vi "Moving Average.vi"(0 "Memory In":refnum<k21>="Running Avg Memory", 2 "N (# of Ave Pts 8 max)":i32, 3 "Moving Point Index":i32, 5 "Data IN":fxp<+/-,28,17>, 7 "Channel#":i32) -> (6 "Averaged Data":fxp<+/-,28,17>)   [LabVIEW 2013]
uses:
  <vilib>/rvi/FXPMathLib/FxpDiv/subVIs/nifxpmath_Div_SimConfig.ctl
  <vilib>/rvi/DataTransferAndStorage/Container/Common/niFpgaContainerExecOnDevCompGetState.vi
  <vilib>/rvi/Memory/Memory_Emulation/nirvimemoryFastEmulationFpgaImpl.vi
  <instcachedir>/0/nirvimemoryFastEmulationFpgaImpl_5FBAB50466BC4C939F684F8805638BFC.lvgen/nirvimemoryFastEmulationFpgaImpl_5FBAB50466BC4C939F684F8805638BFC_021.vi
  <vilib>/rvi/DataTransferAndStorage/Container/Common/niFpgaContainerGetUniqueNameForEmu.vi
  <vilib>/rvi/Memory/Memory_Emulation/niFpgaMemoryEmulationCacheClearOnFirstRun.vi
  <vilib>/rvi/Memory/Memory_Emulation/nirvimemoryEmulationManagerCache_MakeExclusive.vi
  <vilib>/rvi/Memory/Memory_Emulation/niFpgaMemoryEmulationValidateCache.vi
  <vilib>/rvi/Memory/Memory_Emulation/nirvimemoryEmulationManagerCache_ReleaseExclusive.vi
  <vilib>/rvi/Memory/Memory_Emulation/nirvimemoryEmulationManagerCache_InsertValue.vi
  <vilib>/Utility/error.llb/Clear Errors.vi
  <vilib>/rvi/Emulation/niFpgaSctlEmulationGetInTimedLoop.vi
  <vilib>/rvi/Memory/Memory_Emulation/nirvimemoryEmulationManagerCache_SetValue.vi
  <vilib>/rvi/Emulation/niFpgaSctlEmulationResourceMgr.vi
  <vilib>/rvi/Memory/Memory_Emulation/nirvimemoryEmulationManagerCache_GetValue.vi
  <vilib>/rvi/FXPMathLib/FxpDiv/simVIs/DllFxpDivTemp_sub.vi
  <vilib>/rvi/DataTransferAndStorage/Container/XNode/niFpgaContainer.xnode
  <vilib>/rvi/Memory/Memory_Emulation/niFpgaMemoryEmulationRefIn.vi
  <vilib>/rvi/FXPMathLib/FxpDiv/XNode/nifxpmath_Div.xnode
  <vilib>/rvi/FXPMathLib/FxpAdd/XNode/nifxpmath_Add.xnode
  <vilib>/rvi/FXPMathLib/sim/FxpSim.dll
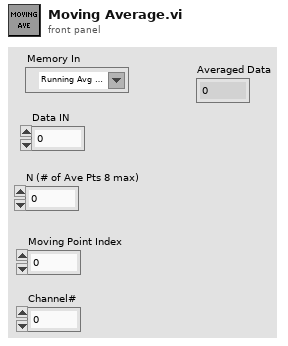
[diagram p1: front panel]
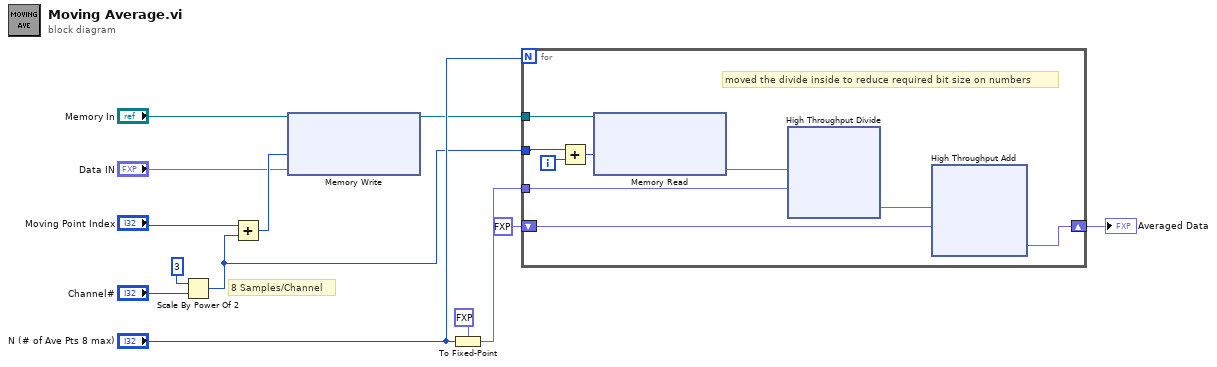
[diagram p0: block diagram]
diagram:
  # "8 Samples/Channel"
  n1 = Scale By Power Of 2(n=i16 3, x="Channel#") -> (x*2^n=w12:i32)
  n2 = Add(x="Moving Point Index", y=w12) -> (x+y=w10:i32)
  n3 = xnode ("Memory Write")("Address"=w10, "Data"="Data IN", "Memory In"="Memory In") -> ("Memory Out"=w11:refnum<k21>)
  n4 = To Fixed-Point(fixed-point type=fxp<+,4,4> 0.0 ("Data IN"), number="N (# of Ave Pts 8 max)") -> (fixed-point=w1:fxp<+,4,4>)
  n5 = for {
    N: "N (# of Ave Pts 8 max)" -> [_]
    tunnel: w11 -> [w20]
    tunnel: w12 -> [w22]
    shift-right: [w17] -> w2
    shift-left: fxp<+/-,26,15> 0.0 ("Data IN") -> [w18]
    tunnel: w1 -> [w15]
    i -> [w21]
    # "moved the divide inside to reduce required bit size on numbers"
    n6 = Add(x=w22, y=w21) -> (x+y=w19:i32)
    n7 = xnode ("Memory Read")("Address"=w19, "Memory In"=w20) -> ("Data"=w16:fxp<+/-,28,17>)  [unwired: 1 out]
    n8 = xnode "High Throughput Divide"("x"=w16, "y"=w15) -> ("x/y"=w14:fxp<+/-,28,17>)
    n9 = xnode ("High Throughput Add")("x"=w14, "y"=w18) -> ("x+y"=w17:fxp<+/-,28,17>)
  }
  "Averaged Data" <- w2
